vi "Begin.vi"(8 "error in":errorcluster) -> (0 "error out":errorcluster)   [LabVIEW 2016]
doc: "Called before other user functions, this VI is expected to open initial I/O refnums, load in file data, and do all program initialization. Notice that the <B>error out</B> terminal is simply used for data flow. Wiring it to other structures or subVIs ensures that this VI runs first."
uses:
  <vilib>/Rock Robotics/WPI/DriverStation/WPI_DriverStationRobotMode2.ctl
  <vilib>/Rock Robotics/WPI/Joystick/WPI_JoystickDeviceEnum.ctl
  <vilib>/Rock Robotics/WPI/ThirdParty/CanMotor/TalonSRX/WPI_CANTalonSRX_APIControlMode.ctl
  <vilib>/Rock Robotics/WPI/Solenoid/WPI_SolenoidChannel.ctl
  Robot Global Data.vi
  <vilib>/Rock Robotics/Network Tables/NT Write String Array.vi
  <vilib>/Rock Robotics/WPI/Solenoid/WPI_SolenoidOpenSingle.vi
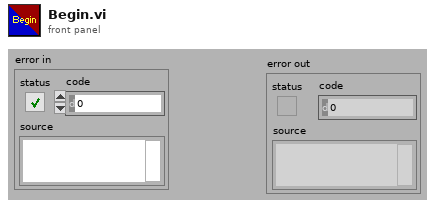
[diagram p1: front panel]
types:
  T1 = typedef "WPI_JoystickDeviceEnum.ctl" = enum16{"USB 0", "USB 1", "USB 2", "USB 3", "USB 4", "USB 5"}
  T2 = typedef "WPI_SolenoidChannel.ctl" = enum8{"Solenoid 0", "Solenoid 1", "Solenoid 2", "Solenoid 3", "Solenoid 4", "Solenoid 5", "Solenoid 6", "Solenoid 7", "Invalid"}
  T3 = typedef "WPI_CANTalonSRX_APIControlMode.ctl" = enum8{"Percent VBus", "Speed", "Position", "Slave", "Unchanged / Invalid", "Voltage Compensation", "Current", "Motion Profile", "Motion Magic"}
  T4 = typedef "WPI_DriverStationRobotMode2.ctl" = enum16{"Autonomous Disabled", "Autonomous Enabled", "Teleop Disabled", "Teleop Enabled", "Disconnected", "Finish", "Test Disabled", "Test Enabled", "Emergency Stopped"}
  T5 = typedef "WPI_JoystickDevRef.ctl" = cluster{"Device":T1}
  T6 = typedef "WPI_MotorControlDeviceRef.ctl" = cluster{"DeviceStatus":errorcluster, "Type":T7, "PWM":cluster{"PWM Channel":T8, "DeadBand":T9}, "CAN":cluster{"Device Number":u8, "SetOutput VI Ref":variant, "GetOutput VI Ref":variant, "Enable VI Ref":variant, "Disable VI Ref":variant, "Data":variant}, "Invert":bool}
  T7 = typedef "WPI_MotorControlType.ctl" = enum16{"PWM", "CAN"}
  T8 = typedef "FPGA_DIOPWMChannel.ctl" = enum8{"PWM 0", "PWM 1", "PWM 2", "PWM 3", "PWM 4", "PWM 5", "PWM 6", "PWM 7", "PWM 8", "PWM 9", "PWM MXP 0", "PWM MXP 1", "PWM MXP 2", "PWM MXP 3", "PWM MXP 4", "PWM MXP 5", "PWM MXP 6", "PWM MXP 7", "PWM MXP 8", "PWM MXP 9", "Invalid"}
  T9 = typedef "WPI_PWMDeadband.ctl" = cluster{"Name":string, "maxPositivePwm":i32, "minPositivePwm":i32, "centerPwm":i32, "maxNegativePwm":i32, "minNegativePwm":i32, "angularRange":u16}
  T10 = typedef "WPI_SolenoidDevRef.ctl" = cluster{"DevStatus":errorcluster, "Pneumatics Control Module":u8, "Forward Solenoid Channel":T2, "Reverse Solenoid Channel":T2}
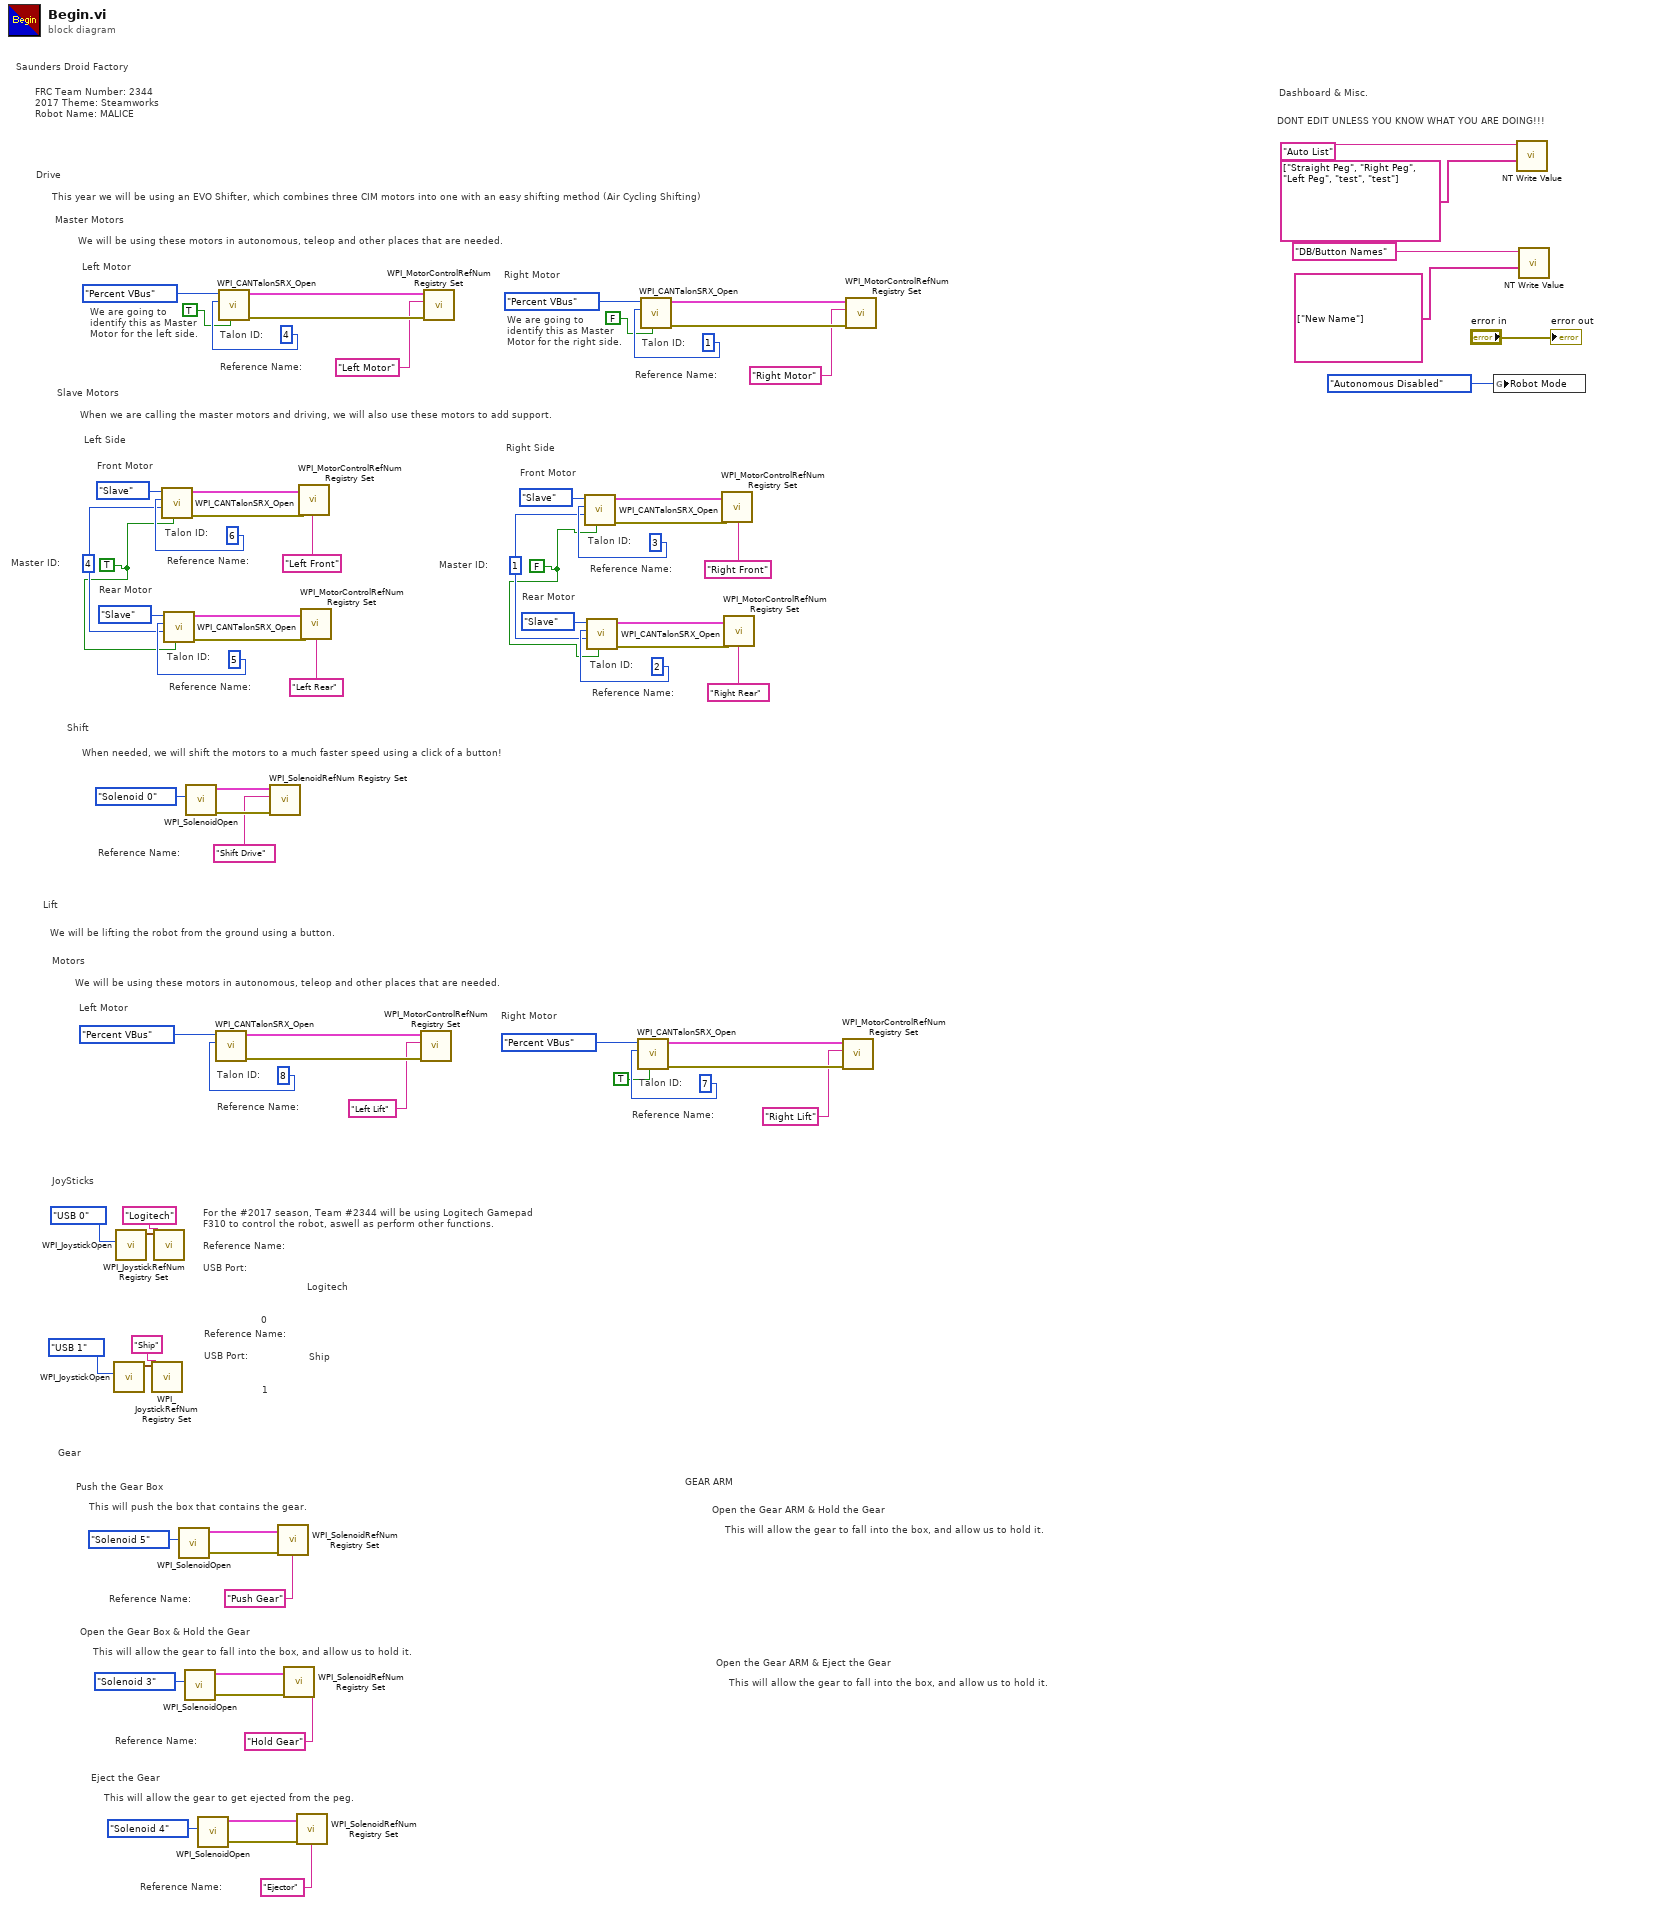
[diagram p0: block diagram]
diagram:
  w19 = TRUE
  w20 = FALSE
  w35 = u8 1 ("Device Number")
  w36 = u8 4 ("Device Number")
  # "This will allow the gear to fall into the box, and allow us to hold it."
  # "Open the Gear ARM & Eject the Gear"
  # "This will allow the gear to fall into the box, and allow us to hold it."
  # "Open the Gear ARM & Hold the Gear"
  # "GEAR ARM"
  # "This will allow the gear to get ejected from the peg."
  # "Eject the Gear"
  # "This will allow the gear to fall into the box, and allow us to hold it."
  # "Open the Gear Box & Hold the Gear"
  # "This will push the box that contains the gear."
  # "Push the Gear Box"
  # "Ship"
  # "1"
  # "Reference Name: \n\nUSB Port:"
  # "Reference Name:"
  # "Reference Name:"
  # "Reference Name:"
  # "DONT EDIT UNLESS YOU KNOW WHAT YOU ARE DOING!!!"
  # "Dashboard & Misc."
  # "Gear"
  # "Reference Name:"
  # "Talon ID:"
  # "Right Motor"
  # "Reference Name:"
  # "Talon ID:"
  # "Left Motor"
  # "We will be using these motors in autonomous, teleop and other places that are needed."
  # "Motors"
  # "We will be lifting the robot from the ground using a button."
  # "Reference Name:"
  # "When needed, we will shift the motors to a much faster speed using a click of a button!"
  # "Shift"
  # "Master ID:"
  # "Master ID:"
  # "Rear Motor"
  # "Reference Name:"
  # "Talon ID:"
  # "Front Motor"
  # "Reference Name:"
  # "Talon ID:"
  # "Rear Motor"
  # "Reference Name:"
  # "Talon ID:"
  # "Front Motor"
  # "Right Side"
  # "Reference Name:"
  # "Talon ID:"
  # "Left Side"
  # "When we are calling the master motors and driving, we will also use these motors to add support."
  # "Slave Motors"
  # "Reference Name:"
  # "Talon ID:"
  # "We are going to \nidentify this as Master Motor for the right side."
  # "Right Motor"
  # "Reference Name:"
  # "Talon ID:"
  # "We are going to \nidentify this as Master Motor for the left side."
  # "Left Motor"
  # "This year we will be using an EVO Shifter, which combines three CIM motors into one with an easy shifting method (Air Cycling Shifting)"
  # "We will be using these motors in autonomous, teleop and other places that are needed."
  # "Master Motors"
  # "JoySticks"
  # "Lift"
  # "Drive"
  # "FRC Team Number: 2344\n2017 Theme: Steamworks\nRobot Name: MALICE"
  # "Saunders Droid Factory"
  # "0"
  # "Logitech"
  # "For the #2017 season, Team #2344 will be using Logitech Gamepad F310 to control the robot, aswell as perform other functions.\n\nReference Name: \n\nUSB Port:"
  n1 = call <vilib>:"WPI_JoystickOpen.vi"("JoystickDevice"=WPI_JoystickDeviceEnum."USB 1") -> ("JoystickDevRef"=w2:T5)  [unwired: 10 in]
  n2 = call <vilib>:"WPI_JoystickOpen.vi"("JoystickDevice"=WPI_JoystickDeviceEnum."USB 0") -> ("JoystickDevRef"=w68:T5)  [unwired: 10 in]
  n3 = call <vilib>:"WPI_JoystickRefNum Registry Set.vi"("refnum name"="Ship", "JoystickDevRef"=w2) -> ()  [unwired: 8 in, 2 out]
  n4 = call <vilib>:"WPI_JoystickRefNum Registry Set.vi"("refnum name"="Logitech", "JoystickDevRef"=w68) -> ()  [unwired: 8 in, 2 out]
  n5 = call <vilib>:"WPI_CANTalonSRX_Open.vi"("Invert"=w19, "Master Device Number"=w36, "Device Number"=u8 6, "Control Mode"=WPI_CANTalonSRX_APIControlMode."Slave") -> ("error out"=w52:errorcluster, "CAN Talon SRX Ref"=w53:T6)  [unwired: 6 in]
  n6 = call <vilib>:"WPI_CANTalonSRX_Open.vi"("Invert"=w19, "Master Device Number"=w36, "Device Number"=u8 5, "Control Mode"=WPI_CANTalonSRX_APIControlMode."Slave") -> ("error out"=w47:errorcluster, "CAN Talon SRX Ref"=w48:T6)  [unwired: 6 in]
  n7 = call-poly <vilib>:"WPI_SolenoidOpen.vi"("Solenoid Channel"=WPI_SolenoidChannel."Solenoid 5") -> ("error out"=w12:errorcluster, "SolenoidDevRef"=w14:T10)  [unwired: 9 in]
  n8 = call-poly <vilib>:"WPI_SolenoidOpen.vi"("Solenoid Channel"=WPI_SolenoidChannel."Solenoid 3") -> ("error out"=w8:errorcluster, "SolenoidDevRef"=w10:T10)  [unwired: 9 in]
  n9 = call-poly <vilib>:"WPI_SolenoidOpen.vi"("Solenoid Channel"=WPI_SolenoidChannel."Solenoid 0") -> ("error out"=w33:errorcluster, "SolenoidDevRef"=w32:T10)  [unwired: 9 in]
  n10 = call-poly <vilib>:"WPI_SolenoidOpen.vi"("Solenoid Channel"=WPI_SolenoidChannel."Solenoid 4") -> ("error out"=w4:errorcluster, "SolenoidDevRef"=w6:T10)  [unwired: 9 in]
  n11 = call <vilib>:"WPI_CANTalonSRX_Open.vi"("Device Number"=u8 8, "Control Mode"=WPI_CANTalonSRX_APIControlMode."Percent VBus") -> ("error out"=w29:errorcluster, "CAN Talon SRX Ref"=w28:T6)  [unwired: 8 in]
  n12 = call <vilib>:"WPI_CANTalonSRX_Open.vi"("Invert"=TRUE, "Device Number"=u8 4, "Control Mode"=WPI_CANTalonSRX_APIControlMode."Percent VBus") -> ("error out"=w64:errorcluster, "CAN Talon SRX Ref"=w63:T6)  [unwired: 7 in]
  n13 = call <vilib>:"WPI_SolenoidRefNum Registry Set.vi"("error in (no error)"=w33, "refnum name"="Shift Drive", "SolenoidDevRef"=w32) -> ()  [unwired: 7 in, 2 out]
  n14 = call <vilib>:"WPI_SolenoidRefNum Registry Set.vi"("error in (no error)"=w12, "refnum name"="Push Gear", "SolenoidDevRef"=w14) -> ()  [unwired: 7 in, 2 out]
  n15 = call <vilib>:"WPI_SolenoidRefNum Registry Set.vi"("error in (no error)"=w8, "refnum name"="Hold Gear", "SolenoidDevRef"=w10) -> ()  [unwired: 7 in, 2 out]
  n16 = call <vilib>:"WPI_SolenoidRefNum Registry Set.vi"("error in (no error)"=w4, "refnum name"="Ejector", "SolenoidDevRef"=w6) -> ()  [unwired: 7 in, 2 out]
  n17 = call <vilib>:"WPI_MotorControlRefNum Registry Set.vi"("error in (no error)"=w52, "refnum name"="Left Front", "MotorControlDevRef"=w53) -> ()  [unwired: 7 in, 2 out]
  n18 = call <vilib>:"WPI_MotorControlRefNum Registry Set.vi"("error in (no error)"=w47, "refnum name"="Left Rear", "MotorControlDevRef"=w48) -> ()  [unwired: 7 in, 2 out]
  n19 = call <vilib>:"WPI_MotorControlRefNum Registry Set.vi"("error in (no error)"=w29, "refnum name"="Left Lift", "MotorControlDevRef"=w28) -> ()  [unwired: 7 in, 2 out]
  n20 = call <vilib>:"WPI_MotorControlRefNum Registry Set.vi"("error in (no error)"=w64, "refnum name"="Left Motor", "MotorControlDevRef"=w63) -> ()  [unwired: 7 in, 2 out]
  n21 = call <vilib>:"WPI_CANTalonSRX_Open.vi"("Invert"=w20, "Master Device Number"=w35, "Device Number"=u8 3, "Control Mode"=WPI_CANTalonSRX_APIControlMode."Slave") -> ("error out"=w42:errorcluster, "CAN Talon SRX Ref"=w43:T6)  [unwired: 6 in]
  n22 = call <vilib>:"WPI_CANTalonSRX_Open.vi"("Invert"=w20, "Master Device Number"=w35, "Device Number"=u8 2, "Control Mode"=WPI_CANTalonSRX_APIControlMode."Slave") -> ("error out"=w37:errorcluster, "CAN Talon SRX Ref"=w38:T6)  [unwired: 6 in]
  n23 = call <vilib>:"WPI_CANTalonSRX_Open.vi"("Invert"=TRUE, "Device Number"=u8 7, "Control Mode"=WPI_CANTalonSRX_APIControlMode."Percent VBus") -> ("error out"=w24:errorcluster, "CAN Talon SRX Ref"=w23:T6)  [unwired: 7 in]
  n24 = call <vilib>:"WPI_CANTalonSRX_Open.vi"("Invert"=FALSE, "Device Number"=u8 1, "Control Mode"=WPI_CANTalonSRX_APIControlMode."Percent VBus") -> ("error out"=w59:errorcluster, "CAN Talon SRX Ref"=w58:T6)  [unwired: 7 in]
  n25 = call <vilib>:"WPI_MotorControlRefNum Registry Set.vi"("error in (no error)"=w42, "refnum name"="Right Front", "MotorControlDevRef"=w43) -> ()  [unwired: 7 in, 2 out]
  n26 = call <vilib>:"WPI_MotorControlRefNum Registry Set.vi"("error in (no error)"=w37, "refnum name"="Right Rear", "MotorControlDevRef"=w38) -> ()  [unwired: 7 in, 2 out]
  n27 = call <vilib>:"WPI_MotorControlRefNum Registry Set.vi"("error in (no error)"=w24, "refnum name"="Right Lift", "MotorControlDevRef"=w23) -> ()  [unwired: 7 in, 2 out]
  n28 = call <vilib>:"WPI_MotorControlRefNum Registry Set.vi"("error in (no error)"=w59, "refnum name"="Right Motor", "MotorControlDevRef"=w58) -> ()  [unwired: 7 in, 2 out]
  n29 = global write "Robot Global Data.vi" "Robot Mode"(WPI_DriverStationRobotMode2."Autonomous Disabled" ("Robot Mode")) -> ()
  n30 = call-poly <vilib>:"NT Write Value.vi"("String Array"=string[] ["Straight Peg", "Right Peg", "Left Peg", "test", "test"], "Name"="Auto List") -> ()  [unwired: 9 in, 1 out]
  n31 = call-poly <vilib>:"NT Write Value.vi"("String Array"=string[] ["New Name"], "Name"="DB/Button Names") -> ()  [unwired: 9 in, 1 out]
  "error out" <- "error in"
